vi "Read settledIsTrue.vi"(11 "SystemController in":refnum<class "SystemController.lvclass">) -> (2 "settledIsTrue":bool, 3 "SystemController out":refnum<class "SystemController.lvclass">)   [LabVIEW 2015, in "SystemController.lvclass"]
uses:
  SystemController.lvclass
  SystemController.lvclass/SystemController.ctl
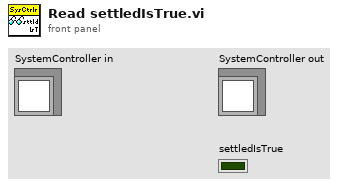
[diagram p1: front panel]
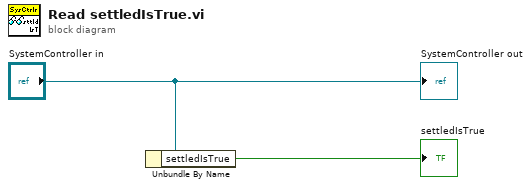
[diagram p0: block diagram]
diagram:
  n1 = Unbundle By Name("SystemController in") -> ("settledIsTrue"=→"settledIsTrue":bool)
  "SystemController out" <- "SystemController in"
